vi "Filter Paths.vi"(7 "Argument":string, 11 "Paths":path[](array[path])) -> (3 "Filtered Path":path[](array[path]))   [LabVIEW 2020, in "VI Properties Editor.lvlib"]
uses:
  VI Properties Editor.lvlib
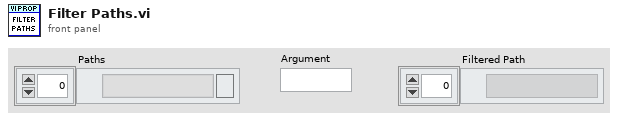
[diagram p1: front panel]
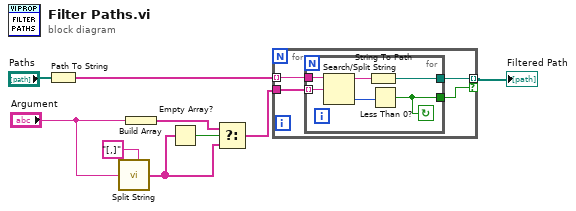
[diagram p0: block diagram]
diagram:
  n1 = Path To String(path="Paths") -> (string=w8:string[])
  n2 = call <vilib>:"Split String.vi"("Split Pattern"="[,]", "Input String"="Argument") -> ("Split String"=w1:string[])  [unwired: 5 in]
  n3 = Build Array("Argument") -> (w2:string[])
  n4 = Empty Array?(array=w1) -> (empty?=w4:bool)
  n5 = Select(t=w2, s=w4, f=w1) -> (s? t:f=w5:string[])
  n6 = for {
    tunnel: w8 -> [w13] mode=indexing
    tunnel: [w11] -> w9 mode=indexing if=w12
    tunnel: w5 -> [w10]
    n7 = for {
      tunnel: w13 -> [w19]
      tunnel: [w14] -> w12
      tunnel: [w16] -> w11
      tunnel: w10 -> [w15] mode=indexing
      stop <- w14 continue-if-true
      n8 = Search/Split String(string=w19, search string/char (-)=w15) -> (substring before match=w18:string, offset of match=w17:i32)  [unwired: 1 in, 1 out]
      n9 = String To Path(string=w18) -> (path=w16:path)
      n10 = Less Than 0?(x=w17) -> (x < 0?=w14:bool)
    }
  }
  "Filtered Path" <- w9
